vi "Shutdown.vi"(8 "error in (no error)":errorcluster, 11 "Optical Spectrum Analyzer In":refnum<class "Optical Spectrum Analyzer.lvclass">) -> (0 "error out":errorcluster, 3 "Optical Spectrum Analyzer Out":refnum<class "Optical Spectrum Analyzer.lvclass">)   [LabVIEW 2018, in "Optical Spectrum Analyzer.lvlib" / "Optical Spectrum Analyzer.lvclass"]
uses:
  Optical Spectrum Analyzer.lvclass
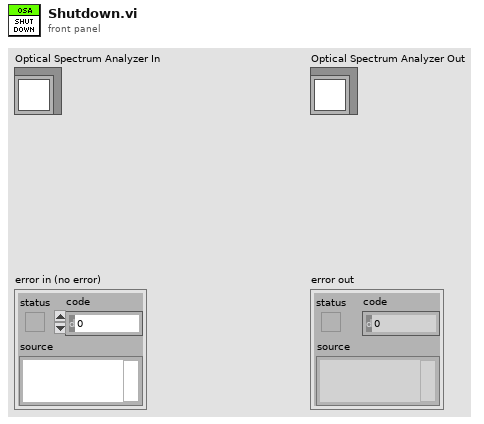
[diagram p1: front panel]
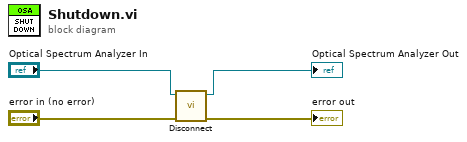
[diagram p0: block diagram]
diagram:
  n1 = call-dynamic "Disconnect.vi"("error in (no error)"="error in (no error)", "Optical Spectrum Analyzer in"="Optical Spectrum Analyzer In") -> ("error out"=→"error out":errorcluster, "Optical Spectrum Analyzer out"=→"Optical Spectrum Analyzer Out":refnum<class "Optical Spectrum Analyzer.lvclass">)  [unwired: 8 in]
